vi "Util_Progress Show Progress Popup.vi"(8 "error in (no error)":errorcluster, 9 "Title":string, 10 "Message":string) -> (0 "error out":errorcluster)   [LabVIEW 2020]
panel:
  out "appended path":path
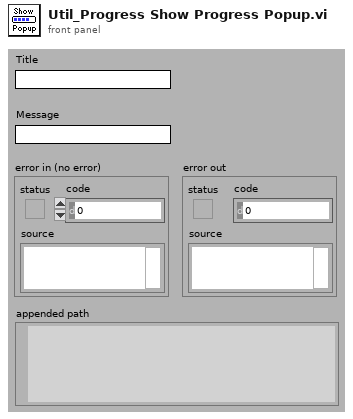
[diagram p1: front panel]
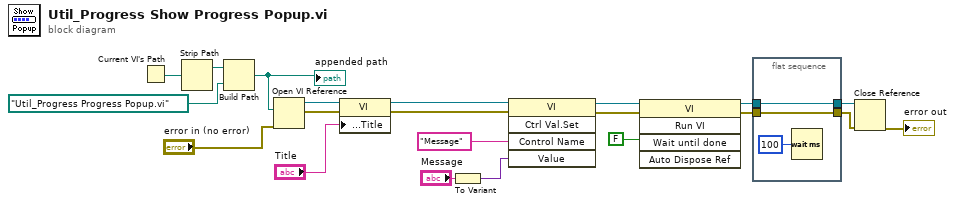
[diagram p0: block diagram]
diagram:
  n1 = Current VI's Path() -> (path=w11:path)
  n2 = Strip Path(path=w11) -> (stripped path=w10:path)  [unwired: 1 out]
  n3 = Build Path(base path=w10, name or relative path=path "Util_Progress Progress Popup.vi" ("vi path")) -> (appended path=w8:path)
  "appended path" <- w8
  n4 = Open VI Reference(vi path=w8, error in (no error)="error in (no error)") -> (vi reference=w20:refnum<vi>, error out=w21:errorcluster)  [unwired: 4 out]
  n5 = property class="VI"(reference=w20, error in=w21, "Front Panel.Title"="Title") -> (reference out=w15:refnum<vi>, error out=w16:errorcluster)
  n6 = To Variant(anything="Message") -> (Variant=w1:variant)
  n7 = invoke class="VI" method="Ctrl Val.Set"(reference=w15, error in=w16, "Control Name"="Message", "Value"=w1) -> (reference out=w2:refnum<vi>, error out=w3:errorcluster)  [unwired: 1 in, 3 out]
  n8 = invoke class="VI" method="Run VI"(reference=w2, error in=w3, "Wait until done"=FALSE ("Wait Until Done")) -> (reference out=w7:refnum<vi>, error out=w5:errorcluster)  [unwired: 2 in, 3 out]
  n9 = flat-sequence {
    tunnel: [w24] -> w6
    tunnel: w7 -> [w24]
    tunnel: [w23] -> w4
    tunnel: w5 -> [w23]
    frame #0 {
      n10 = Wait (ms)(milliseconds to wait=u32 100) -> ()  [unwired: 1 out]
    }
  }
  n11 = Close Reference(reference=w6, error in (no error)=w4) -> (error out=→"error out":errorcluster)
